vi "Run.vi"(8 "error in (no error)":errorcluster, 9 "s on last turn":dbl, 10 "Maze (0: Empty, -1: Enemy. >0: Teammate":i32[][](array[numeric]), 11 "Spawn in":refnum<class "Spawn.lvclass">) -> (0 "error out":errorcluster, 1 "Direction":T1, 2 "Action":T2, 3 "Spawn out":refnum<class "Spawn.lvclass">, 4 "Replicated":refnum<class "Square.lvclass">)   [LabVIEW 2015, in "Spawn.lvclass"]
uses:
  Spawn.lvclass
  Type Defs/Action Enum.ctl
  Type Defs/Direction Enum.ctl
  Square/Square.lvclass
  Spawn.lvclass/Spawn.ctl
  Attack/Attack.lvclass
  Attack/Attack.lvclass/Attack.ctl
  Attack/Write Deviation.vi
  Attack/Write Direction.vi
  Attack/Write Frequency.vi
  SubVIs/Read-Only Globals.vi
  Type Defs/SB Type Defs.lvlib
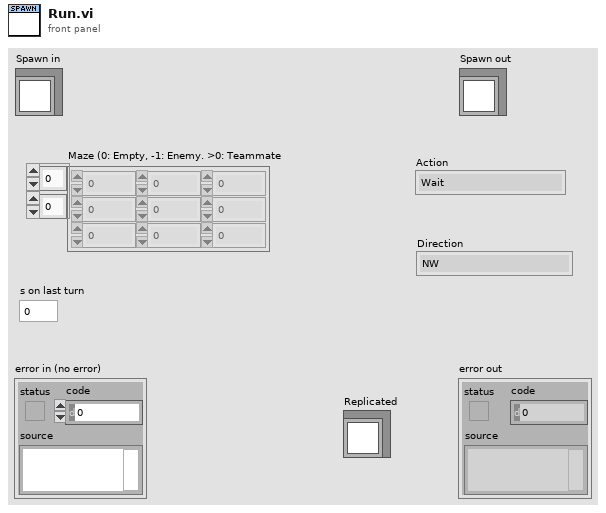
[diagram p1: front panel]
types:
  T1 = typedef "SB Type Defs.lvlib/Direction Enum.ctl" = enum16{"NW", "N", "NE", "E", "SE", "S", "SW", "W"}
  T2 = typedef "SB Type Defs.lvlib/Action Enum.ctl" = enum16{"Wait", "Move", "Attack", "Replicate"}
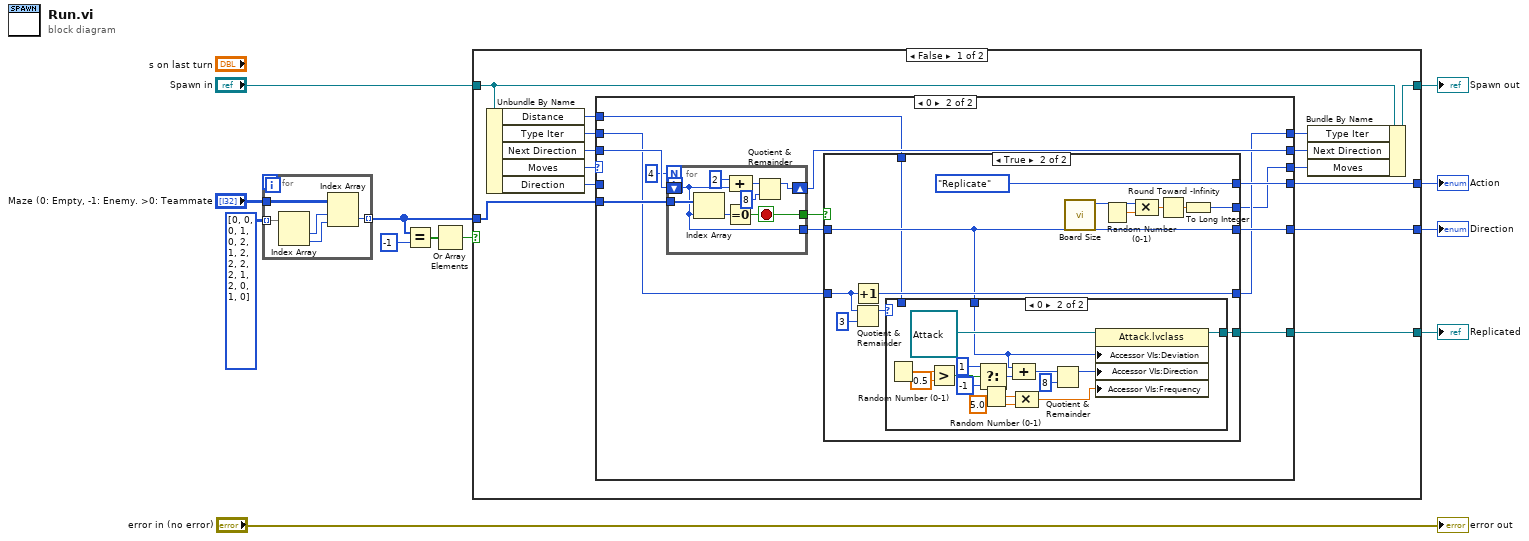
[diagram p0: block diagram]
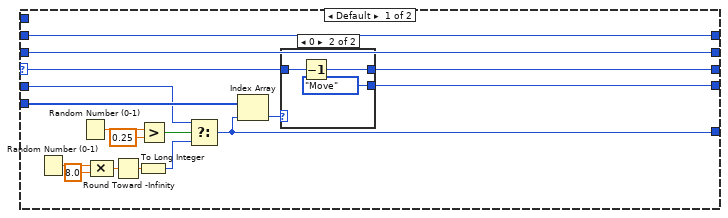
[diagram p2: hidden frame]
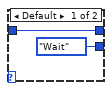
[diagram p3: hidden frame]
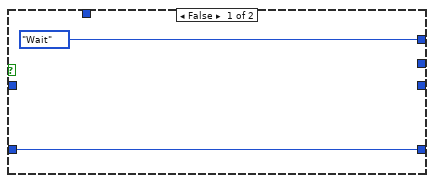
[diagram p4: hidden frame]
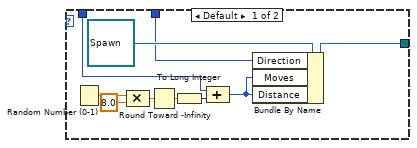
[diagram p5: hidden frame]
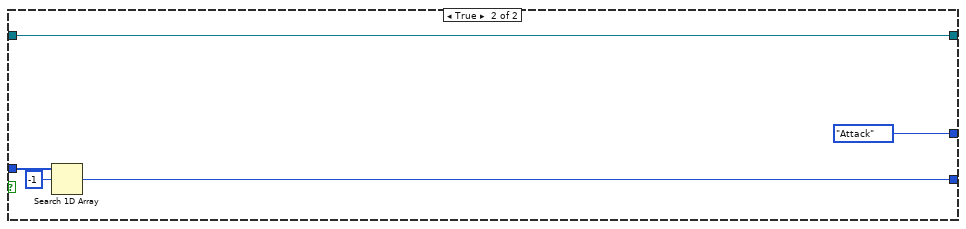
[diagram p6: hidden frame]
diagram:
  n1 = for {
    tunnel: "Maze (0: Empty, -1: Enemy. >0: Teammate" -> [w17]
    tunnel: i32[][] [[0, 0], [0, 1], [0, 2], [1, 2], [2, 2], [2, 1], [2, 0], [1, 0]] -> [w16] mode=indexing
    tunnel: [w13] -> w4 mode=indexing
    n2 = Index Array(array=w16) -> (element #1=w15:i32, element #2=w14:i32)  [unwired: 2 in]
    n3 = Index Array(array=w17, index (row)=w15, index (col)=w14) -> (element=w13:i32)
  }
  n4 = Equal?(x=w4, y=-1) -> (x = y?=w3:bool[])
  n5 = Or Array Elements(Boolean array=w3) -> (logical OR=w2:bool)
  n6 = case shown="False" w2 {
    tunnel: [w31 Action_Enum."Attack" ("Action")] -> w11
    tunnel: "Spawn in" -> [w29 w119]
    tunnel: [w28 w119] -> w10
    tunnel: [w26 w115] -> w9
    tunnel: [w24 _] -> w8
    tunnel: w4 -> [w21 w117]
    frame False {
      n7 = Unbundle By Name(w29) -> ("Distance"=w18:i32, "Type Iter"=w20:i32, "Next Direction"=w23:T1, "Moves"=w30:i32, "Direction"=w25:T1)
      n8 = case shown="0" w30 {
        selector: w30 -> [w48 _]
        tunnel: [w46 w66] -> w31
        tunnel: [w47 w54] -> w27
        tunnel: w25 -> [w33 _]
        tunnel: [w32 w65] -> w26
        tunnel: [_ w64] -> w24
        tunnel: w23 -> [w44 w63]
        tunnel: [w44 w62] -> w22
        tunnel: w21 -> [w43 w61]
        tunnel: w20 -> [w42 w60]
        tunnel: [w42 w59] -> w19
        tunnel: w18 -> [_ w55]
        frame Default {
          n9 = Random Number (0-1)() -> (number: 0 to 1=w39:dbl)
          n10 = Random Number (0-1)() -> (number: 0 to 1=w41:dbl)
          n11 = Compound Arithmetic op=MULTIPLY(w39, 8.0 ("value")) -> (w37:dbl)
          n12 = Round Toward -Infinity(1:w37) -> (0:w35:dbl)
          n13 = To Long Integer(number=w35) -> (32bit integer=w34:i32)
          n14 = Greater?(x=w41, y=0.25) -> (0:w36:bool)
          n15 = Select(t=w33, s=w36, f=w34) -> (s? t:f=w32:i32)
          n16 = Index Array(array=w43, index=w32) -> (element=w45:i32)
          n17 = case shown="0" w45 {
            tunnel: w48 -> [w50 w53]
            tunnel: [w50 w52] -> w47
            tunnel: [Action_Enum."Wait" ("Action") Action_Enum."Move" ("Action")] -> w46
            frame Default {
            }
            frame 0 {
              n18 = Decrement(x=w53) -> (x-1=w52:i32)
            }
          }
        }
        frame 0 {
          n19 = for {
            N: 4 -> [_]
            tunnel: w61 -> [w114]
            tunnel: [w112] -> w57
            shift-right: [w109] -> w62
            shift-left: w63 -> [w107]
            tunnel: [w107] -> w56
            stop <- w112 stop-if-true
            n20 = Index Array(array=w114, index=w107) -> (element=w113:i32)
            n21 = Equal To 0?(x=w113) -> (x = 0?=w112:bool)
            n22 = Compound Arithmetic op=ADD(2, w107) -> (w110:i32)
            n23 = Quotient & Remainder(x=w110, y=8) -> (x-y*floor(x/y)=w109:i32)  [unwired: 1 out]
          }
          n24 = case shown="True" w57 {
            tunnel: [Action_Enum."Wait" ("Action") Action_Enum."Replicate" ("Action")] -> w66
            tunnel: [_ w75] -> w65
            tunnel: w56 -> [_ w75]
            tunnel: w60 -> [w67 w79]
            tunnel: [w67 w78] -> w59
            tunnel: [_ w76] -> w64
            tunnel: w55 -> [_ w74]
            tunnel: [_ w70] -> w54
            frame False {
            }
            frame True {
              n25 = Increment(x=w79) -> (x+1=w78:i32)
              n26 = Quotient & Remainder(x=w79, y=3) -> (x-y*floor(x/y)=w77:i32)  [unwired: 1 out]
              n27 = case shown="0" w77 {
                tunnel: [w90 w105] -> w76
                tunnel: w75 -> [w89 w101]
                tunnel: w74 -> [w82 _]
                frame Default {
                  n28 = Random Number (0-1)() -> (number: 0 to 1=w88:dbl)
                  n29 = Compound Arithmetic op=MULTIPLY(w88, 8.0 ("value")) -> (w86:dbl)
                  n30 = Round Toward -Infinity(1:w86) -> (0:w85:dbl)
                  n31 = To Long Integer(number=w85) -> (32bit integer=w84:i32)
                  n32 = Compound Arithmetic op=ADD(w82, w84) -> (w83:i32)
                  n33 = Bundle By Name(cluster=refnum<class "Spawn.lvclass"> refnum ("Spawn.lvclass"), "Direction"=w89, "Moves"=w83, "Distance"=w83) -> (w90:refnum<class "Spawn.lvclass">)
                }
                frame 0 {
                  n34 = Random Number (0-1)() -> (number: 0 to 1=w104:dbl)
                  n35 = Greater?(x=w104, y=0.5) -> (0:w102:bool)
                  n36 = Select(t=1, s=w102, f=-1) -> (s? t:f=w100:i32)
                  n37 = Random Number (0-1)() -> (number: 0 to 1=w94:dbl)
                  n38 = Compound Arithmetic op=ADD(w101, w100) -> (w97:i32)
                  n39 = Compound Arithmetic op=MULTIPLY(w94, 5.0 ("value")) -> (w92:dbl)
                  n40 = Quotient & Remainder(x=w97, y=8) -> (x-y*floor(x/y)=w96:i32)  [unwired: 1 out]
                  n41 = property class="Attack.lvclass"(reference=refnum<class "Attack.lvclass"> refnum ("Attack.lvclass"), "Accessor VIs:Deviation"=w101, "Accessor VIs:Direction"=w96, "Accessor VIs:Frequency"=w92) -> (reference out=w105:refnum<class "Attack.lvclass">)  [unwired: 1 in, 1 out]
                }
              }
              n42 = call "Board Size.vi"() -> ("Board Size"=w69:i32)  [unwired: 11 in]
              n43 = Random Number (0-1)() -> (number: 0 to 1=w71:dbl)
              n44 = Compound Arithmetic op=MULTIPLY(w69, w71) -> (w72:dbl)
              n45 = Round Toward -Infinity(1:w72) -> (0:w73:dbl)
              n46 = To Long Integer(number=w73) -> (32bit integer=w70:i32)
            }
          }
        }
      }
      n47 = Bundle By Name(cluster=w29, "Type Iter"=w19, "Next Direction"=w22, "Moves"=w27) -> (w28:refnum<class "Spawn.lvclass">)
    }
    frame True {
      n48 = Search 1D Array(1D array=w117, element=-1) -> (index of element=w115:i32)  [unwired: 1 in]
    }
  }
  "Spawn out" <- w10
  "Action" <- w11
  "Direction" <- w9
  "Replicated" <- w8
  "error out" <- "error in (no error)"
